vi "Heading Correction.vi"(2 "Count In":i32, 3 "Current Heading":dbl) -> (0 "Count Out":i32, 1 "Transformed Heading":dbl format="%0.2f")   [LabVIEW 2015]
uses:
  <vilib>/Analysis/baseanly.llb/Mean (DBL).vi
  <vilib>/Analysis/NI_AALBase.lvlib
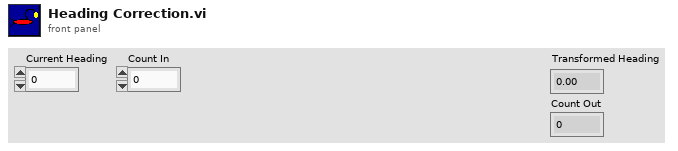
[diagram p1: front panel]
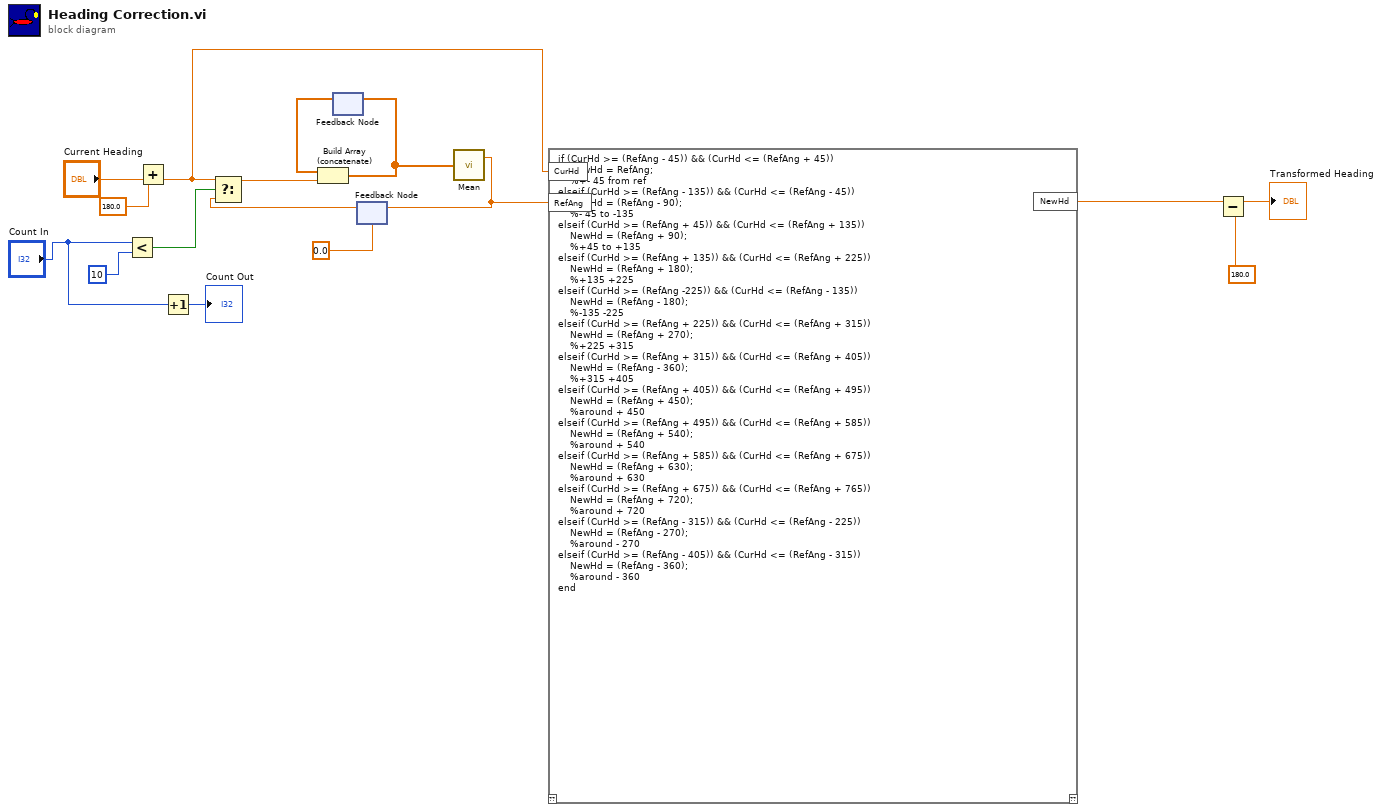
[diagram p0: block diagram]
diagram:
  n1 = Less?(x="Count In", y=10) -> (x < y?=w13:bool)
  n2 = Add(x=180.0, y="Current Heading") -> (x+y=w5:dbl)
  n3 = Increment(x="Count In") -> (x+1=→"Count Out":i32)
  n4 = feedback #1() -> (w16:dbl[])  [unwired: 1 in]
  n5 = feedback #2(0.0 ("mean")) -> (w11:dbl)
  n6 = Select(t=w5, s=w13, f=w11) -> (s? t:f=w14:dbl)
  n7 = Build Array (concatenate)(w16, w14) -> (w12:dbl[])
  n8 = feedback-in #1(w12) -> ()
  n9 = call-poly <vilib>:"Mean.vi"("X"=w12) -> ("mean"=w9:dbl)  [unwired: 1 out]
  n10 = feedback-in #2(w9) -> ()
  n11 = script code="if (CurHd >= (RefAng - 45)) && (CurHd <= (RefAng + 45))\n    NewHd = RefAng;\n    %+- 45 from ref\nelseif (CurHd >= (RefAng - 135)) && (CurHd <= (RefAng - 45))\n    NewHd = (RefAng - 90);\n    %- 45 to -135\nelseif (CurHd >= (RefAng + 45)) && (CurHd <= (RefAng + 135))\n    NewHd = (RefAng + 90);\n    %+45 to +135\nelseif (CurHd >= (RefAng + 135)) && (CurHd <= (RefAng + 225))\n    NewHd = (RefAng + 180);\n    %+135 +225\nelseif (CurHd >= (RefAng -225)) && (CurHd <= (RefAng - 135))\n    NewHd = (RefAng - 180);\n    %-135 -225\nelseif (CurHd >= (RefAng + 225)) && (CurHd <= (RefAng + 315))\n    NewHd = (RefAng + 270);\n    %+225 +315\nelseif (CurHd >= (RefAng + 315)) && (CurHd <= (RefAng + 405))\n    NewHd = (RefAng - 360);\n    %+315 +405\nelseif (CurHd >= (RefAng + 405)) && (CurHd <= (RefAng + 495))\n    NewHd = (RefAng + 450);\n    %around + 450\nelseif (CurHd >= (RefAng + 495)) && (CurHd <= (RefAng + 585))\n    NewHd = (RefAng + 540);\n    %around + 540\nelseif (CurHd >= (RefAng + 585)) && (CurHd <= (RefAng + 675))\n    NewHd = (RefAng + 630);\n    %around + 630\nelseif (CurHd >= (RefAng + 675)) && (CurHd <= (RefAng + 765))\n    NewHd = (RefAng + 720);\n    %around + 720\nelseif (CurHd >= (RefAng - 315)) && (CurHd <= (RefAng - 225))\n    NewHd = (RefAng - 270);\n    %around - 270\nelseif (CurHd >= (RefAng - 405)) && (CurHd <= (RefAng - 315))\n    NewHd = (RefAng - 360);\n    %around - 360\nend"("RefAng"=w9, "CurHd"=w5) -> ("NewHd"=w2:dbl)  [unwired: 1 in, 1 out]
  n12 = Subtract(x=w2, y=180.0) -> (x-y=→"Transformed Heading":dbl)
